vi "Set BuildSpec Source.vi"(7 "BuildSpec Source":T1, 8 "Error In":errorcluster, 9 "Source Index":i32, 10 "Source Item in":refnum<vi>, 11 "Project Sync Tools in":refnum<class "Project Sync Tools.lvclass">) -> (0 "error out":errorcluster, 2 "Source Item out":refnum<vi>, 3 "Project Sync Tools out":refnum<class "Project Sync Tools.lvclass">)   [LabVIEW 2019, in "Project Sync Tools.lvclass"]
uses:
  Project Sync Tools.lvclass
  TypeDefs/Source Parameters.ctl
  Project Sync Tools.lvclass/Project Sync Tools.ctl
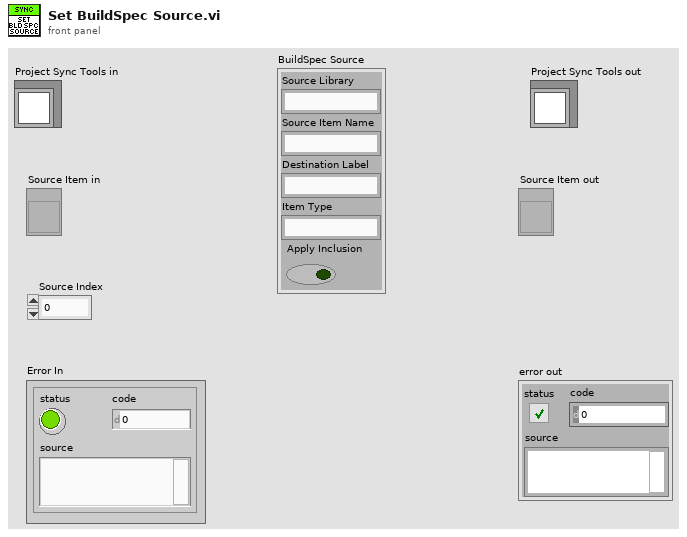
[diagram p1: front panel]
types:
  T1 = typedef "Project Sync Tools.lvclass/Source Parameters.ctl" = cluster{"Source Library":string, "Source Item Name":string, "Destination Label":string, "Item Type":string, "Apply Inclusion":bool}
  T2 = typedef "Project Sync Tools.lvclass/BuildSpec Raw Parameters.ctl" = cluster{"BuildSpec Ref":refnum<vi>, "Target Name":string, "Build Spec Name":string, "Tags":string[], "Tag Values":variant[]}
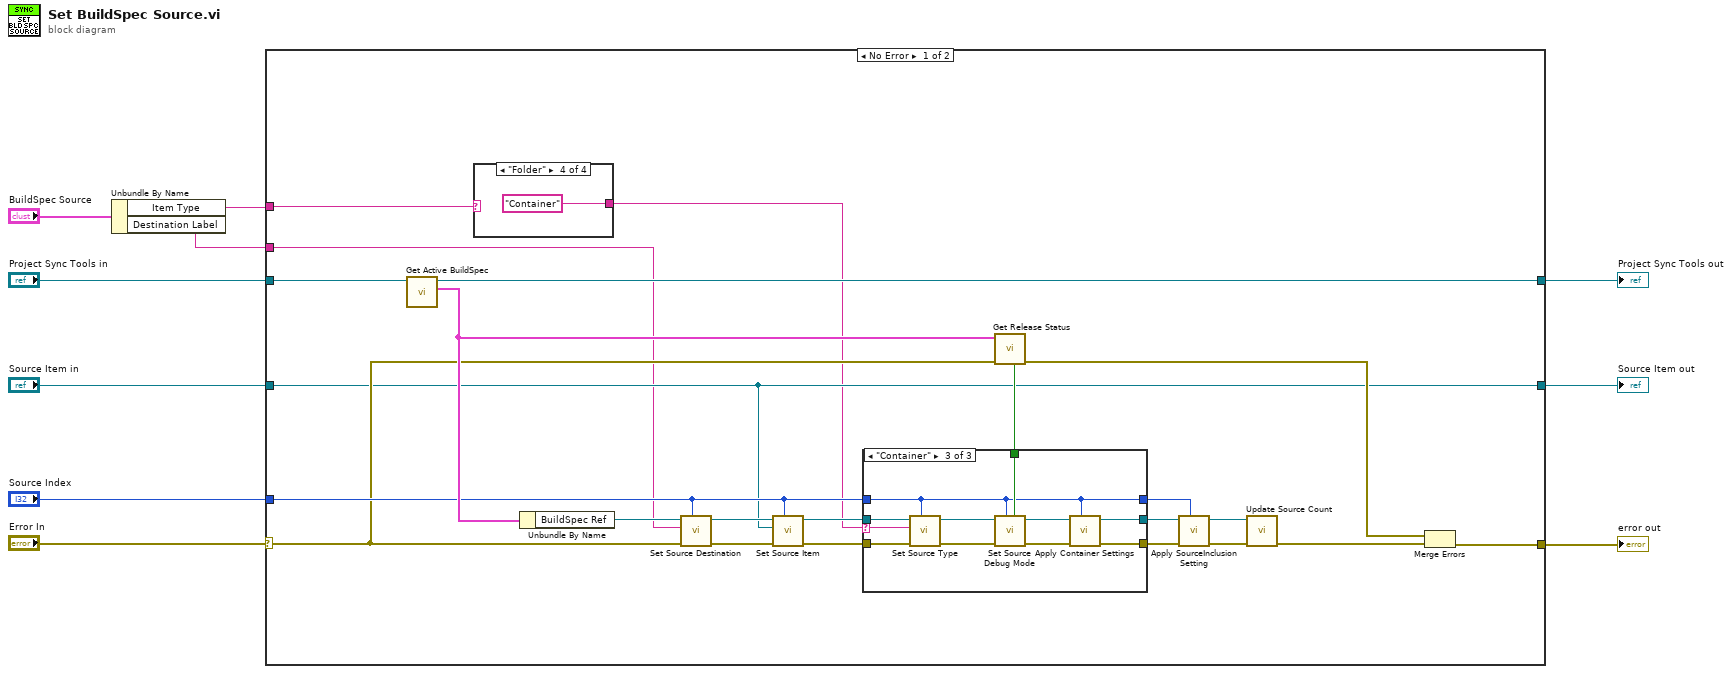
[diagram p0: block diagram]
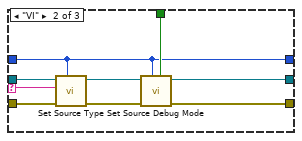
[diagram p3: hidden frame]
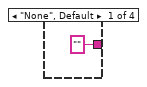
[diagram p4: hidden frame]
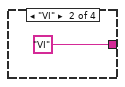
[diagram p5: hidden frame]
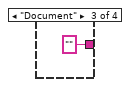
[diagram p6: hidden frame]
diagram:
  n1 = Unbundle By Name("BuildSpec Source") -> ("Item Type"=w2:string, "Destination Label"=w1:string)
  n2 = case shown="No Error" "Error In" {
    selector: "Error In" -> [w22 w63]
    tunnel: "Source Item in" -> [w20 w61]
    tunnel: [w21 w63] -> w9
    tunnel: "Project Sync Tools in" -> [w26 w62]
    tunnel: [w25 w62] -> w7
    tunnel: "Source Index" -> [w23 _]
    tunnel: [w20 w61] -> w4
    tunnel: w2 -> [w19 _]
    tunnel: w1 -> [w18 _]
    frame No Error {
      n3 = call "Get Active BuildSpec.vi"("Project Sync Tools in"=w26) -> ("Build Spec Parameters"=w24:T2, "Project Sync Tools out"=w25:refnum<class "Project Sync Tools.lvclass">)  [unwired: 9 in]
      n4 = case shown="\"Folder\"" w19 {
        tunnel: ["" ("Source Type") "VI" ("Source Type") "" ("Source Type") "Container" ("Source Type")] -> w17
        frame "None", Default {
        }
        frame "VI" {
        }
        frame "Document" {
        }
        frame "Folder" {
        }
      }
      n5 = Unbundle By Name(w24) -> ("BuildSpec Ref"=w27:refnum<vi>)
      n6 = call "Set Source Destination.vi"("Source Index"=w23, "error in (no error)"=w22, "Destination Label"=w18, "BuildSpec in"=w27) -> ("error out"=w32:errorcluster, "BuildSpec out"=w33:refnum<vi>)  [unwired: 6 in]
      n7 = call "Set Source Item.vi"("Source Index"=w23, "error in (no error)"=w32, "Project Item"=w20, "Build Spec in"=w33) -> ("error out"=w31:errorcluster, "Build Spec out"=w30:refnum<vi>)  [unwired: 6 in]
      n8 = call "Get Release Status.vi"("error in"=w22, "Build Spec in"=w24) -> ("error out"=w28:errorcluster, "Is Release"=w29:bool)  [unwired: 7 in, 1 out]
      n9 = case shown="\"Container\"" w17 {
        selector: w17 -> [_ w38 w51]
        tunnel: w31 -> [w34 w45 w56]
        tunnel: w30 -> [w35 w44 w55]
        tunnel: [w34 w41 w48] -> w13
        tunnel: [w35 w40 w47] -> w12
        tunnel: w29 -> [_ w39 w52]
        tunnel: w23 -> [w36 w37 w46]
        tunnel: [w36 w37 w46] -> w11
        frame "None", Default {
        }
        frame "VI" {
          n10 = call "Set Source Type.vi"("Source Index"=w37, "error in (no error)"=w45, "Source Type"=w38, "ProjectItem in"=w44) -> ("error out"=w43:errorcluster, "ProjectItem out"=w42:refnum<vi>)  [unwired: 6 in]
          n11 = call "Set Source Debug Mode.vi"("is Release?"=w39, "Source Index"=w37, "error in (no error)"=w43, "ProjectItem in"=w42) -> ("error out"=w41:errorcluster, "ProjectItem out"=w40:refnum<vi>)  [unwired: 6 in]
        }
        frame "Container" {
          n12 = call "Set Source Type.vi"("Source Index"=w46, "error in (no error)"=w56, "Source Type"=w51, "ProjectItem in"=w55) -> ("error out"=w54:errorcluster, "ProjectItem out"=w53:refnum<vi>)  [unwired: 6 in]
          n13 = call "Set Source Debug Mode.vi"("is Release?"=w52, "Source Index"=w46, "error in (no error)"=w54, "ProjectItem in"=w53) -> ("error out"=w50:errorcluster, "ProjectItem out"=w49:refnum<vi>)  [unwired: 6 in]
          n14 = call "Apply Container Settings.vi"("Source Index"=w46, "error in (no error)"=w50, "BuildSpec in"=w49) -> ("error out"=w48:errorcluster, "BuildSpec out"=w47:refnum<vi>)  [unwired: 7 in]
        }
      }
      n15 = call "Apply SourceInclusion Setting.vi"("Source Index"=w11, "error in (no error)"=w13, "ProjectItem in"=w12) -> ("error out"=w16:errorcluster, "ProjectItem out"=w14:refnum<vi>)  [unwired: 7 in]
      n16 = call "Update Source Count.vi"("error in (no error)"=w16, "BuildSpec in"=w14) -> ("error out"=w15:errorcluster)  [unwired: 8 in, 1 out]
      n17 = Merge Errors(w28, w15) -> (w21:errorcluster)
    }
    frame Error {
    }
  }
  "Project Sync Tools out" <- w7
  "error out" <- w9
  "Source Item out" <- w4
